vi "(SubVI)Serial_Write-Read.vi"(5 "Delay (ms)":u32, 7 "Option":T1, 8 "error in (no error)":errorcluster caption="에러 입력(에러 없음)", 11 "Data to Write":u8[](array[numeric])) -> (0 "error out":errorcluster caption="에러 출력", 2 "Header":T2, 3 "Read Data":u8[](array[numeric]))   [LabVIEW 2020]
uses:
  Controls/(Ctrl)Serial_Protocol Header.ctl
  Controls/(Ctrl)Serial_Write Read Option.ctl
  5cf30121-6025-4447-9d83-457b2d877e1d.vi
  (SubVI)Serial_Write.vi
  (SubVI)Serial_Read.vi
panel:
  # "(SubVI)Serial_Write-Read.vi By hspark\n\nDescription : 시리얼 통신 읽기 동작 후 쓰기 동작을 실행하는 VI\n\nInput : \n1. Data to Write : 쓰기할 데이터 입력\n2. Option : 쓰기 및 읽기 동작 수행 시의 설정 입력\n3. Delay (ms) : 쓰기, 읽기 동작 사이의 Delay 입력\n\nOutput : \n1. Read Data : 읽기한 데이터 출력. Option 중 User Code Verification이 True인 경우 Header를 제외한 앞 2Byte를 제외한 후 출력.\n\nLabVIEW Version : 2020 SP1 이상\n\nNote :\n\nUpdate : 2021.10.06"
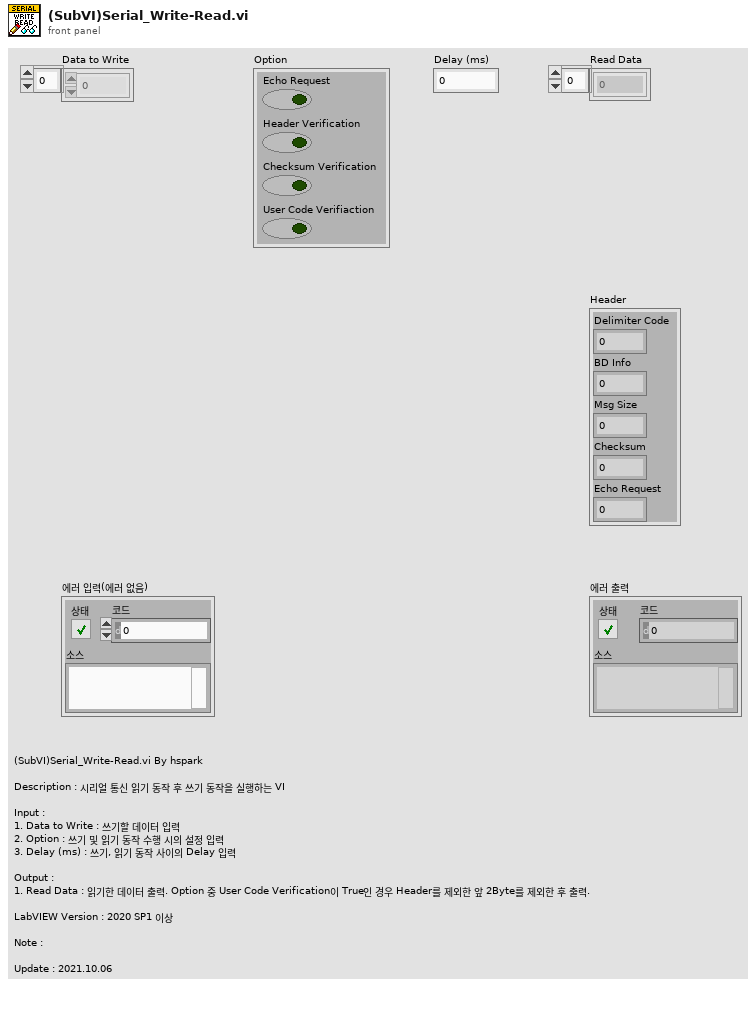
[diagram p1: front panel]
types:
  T1 = typedef "(Ctrl)Serial_Write Read Option.ctl" = cluster{"Echo Request":bool, "Header Verification":bool, "Checksum Verification":bool, "User Code Verifiaction":bool}
  T2 = typedef "(Ctrl)Serial_Protocol Header.ctl" = cluster{"Delimiter Code":u8, "BD Info":u8, "Msg Size":u16, "Checksum":u8, "Echo Request":u8}
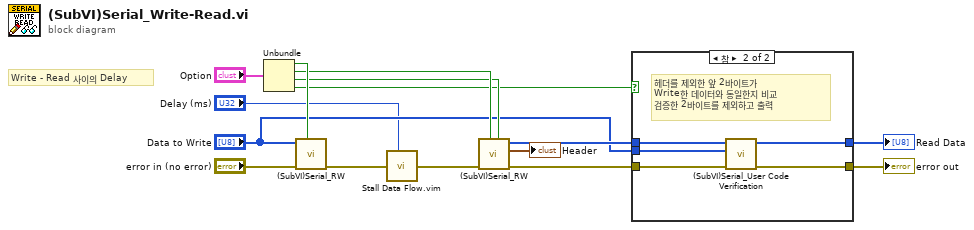
[diagram p0: block diagram]
diagram:
  # "Write - Read 사이의 Delay"
  n1 = Unbundle("Option") -> ("Echo Request"=w11:bool, "Header Verification"=w10:bool, "Checksum Verification"=w9:bool, "User Code Verifiaction"=w4:bool)
  n2 = call-poly "(SubVI)Serial_RW.vi"("Echo Request"=w11, "error in (no error)"="error in (no error)", "Data to Write"="Data to Write") -> ("error out"=w15:errorcluster)  [unwired: 8 in]
  n3 = call "Stall Data Flow.vim"("value in"=w15, "milliseconds to wait"="Delay (ms)") -> ("value out"=w2:errorcluster)  [unwired: 1 out]
  n4 = call-poly "(SubVI)Serial_RW.vi"("Checksum Verification"=w9, "Header Verification"=w10, "error in (no error)"=w2) -> ("error out"=w8:errorcluster, "Header"=→"Header":T2, "Read Data"=w5:u8[])  [unwired: 6 in]
  n5 = case shown="참" w4 {
    tunnel: "Data to Write" -> [_ w22]
    tunnel: [w17 w21] -> w14
    tunnel: w8 -> [w16 w20]
    tunnel: [w16 w19] -> w7
    tunnel: w5 -> [w17 w18]
    frame False {
    }
    frame True {
      # "헤더를 제외한 앞 2바이트가\nWrite한 데이터와 동일한지 비교\n검증한 2바이트를 제외하고 출력"
      n6 = call "(SubVI)Serial_User Code Verification.vi"("에러 입력(에러 없음)"=w20, "Data to Write"=w22, "Read Data"=w18) -> ("에러 출력"=w19:errorcluster, "Read Data"=w21:u8[])  [unwired: 7 in]
    }
  }
  "Read Data" <- w14
  "error out" <- w7
